vi "Test Step Parser.vi"(0 "Controller?":bool, 1 "LastDataTime":i64, 2 "Enum.Radio":enum32{"Flow", "Test", "Hot\nFuel"}(ring)=enum."Test", 5 "Step In":i32, 7 "CMD Cluster IN":T1, 9 "Profile":string[][](array[string]), 11 "Stable Count":dbl format="%#_13g", 12 "Parameter Timeout":dbl format="%#_13g") -> (3 "StepDataActive":dbl, 4 "StepTimeLimit":dbl, 6 "Step Out":i32, 8 "CMD Cluster Out":T1)   [LabVIEW 2019]
uses:
  TypeDef/Command Cluster.ctl
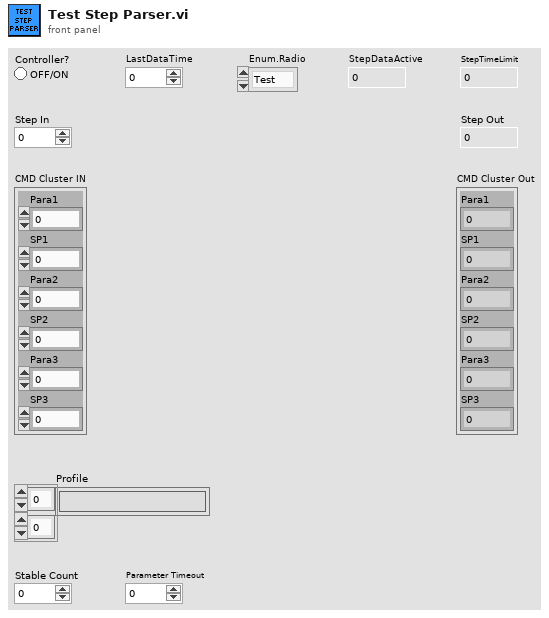
[diagram p1: front panel]
types:
  T1 = typedef "Command Cluster.ctl" = cluster{"Para1":i32, "SP1":dbl, "Para2":i32, "SP2":dbl, "Para3":i32, "SP3":dbl}
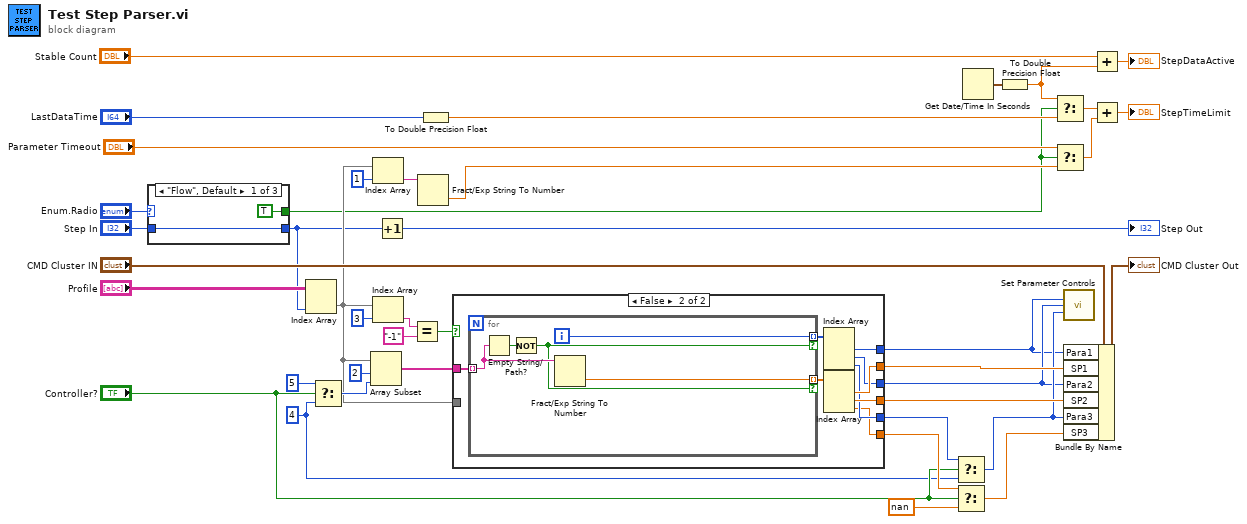
[diagram p0: block diagram]
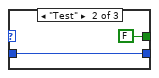
[diagram p2: hidden frame]
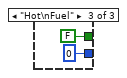
[diagram p3: hidden frame]
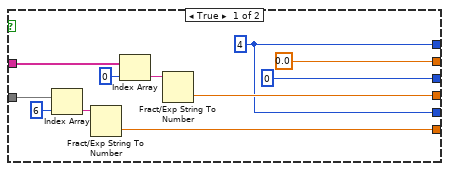
[diagram p4: hidden frame]
diagram:
  w24 = 4 ("index")
  n1 = case shown="\"Flow\", Default" "Enum.Radio" {
    tunnel: [TRUE FALSE FALSE] -> w1
    tunnel: "Step In" -> [w42 w44 _]
    tunnel: [w42 w44 0 ("Step In")] -> w2
    frame "Flow", Default {
    }
    frame "Test" {
    }
    frame "Hot\nFuel" {
    }
  }
  n2 = Index Array(array="Profile", index (col)=w2) -> (element=w19:string[])  [unwired: 1 in]
  n3 = Select(t=5 ("length"), s="Controller?", f=w24) -> (s? t:f=w29:i32)
  n4 = Array Subset(array=w19, index=2, length=w29) -> (w37:string[])
  n5 = Index Array(array=w19, index=1) -> (element=w17:string)
  n6 = Index Array(array=w19, index=3) -> (element=w33:string)
  n7 = Increment(x=w2) -> (x+1=→"Step Out":i32)
  n8 = Equal?(x=w33, y="-1") -> (x = y?=w31:bool)
  n9 = Fract/Exp String To Number(string=w17) -> (number=w13:dbl)  [unwired: 3 in, 1 out]
  n10 = To Double Precision Float(number="LastDataTime") -> (double precision float=w5:dbl)
  n11 = case shown="False" w31 {
    tunnel: w37 -> [w58 w67]
    tunnel: [0.0 w64] -> w36
    tunnel: [w55 w63] -> w35
    tunnel: [w52 w62] -> w20
    tunnel: [0 w61] -> w21
    tunnel: [w52 w60] -> w26
    tunnel: [w48 w59] -> w28
    tunnel: w19 -> [w49 _]
    frame True {
      w52 = 4
      n12 = Index Array(array=w49, index=6) -> (element=w50:string)
      n13 = Fract/Exp String To Number(string=w50) -> (number=w48:dbl)  [unwired: 3 in, 1 out]
      n14 = Index Array(array=w58, index=0) -> (element=w56:string)
      n15 = Fract/Exp String To Number(string=w56) -> (number=w55:dbl)  [unwired: 3 in, 1 out]
    }
    frame False {
      n16 = for {
        tunnel: w67 -> [w72] mode=indexing
        tunnel: [w68] -> w66 mode=indexing if=w69
        tunnel: [w70] -> w65 mode=indexing if=w69
        i -> [w70]
        n17 = Empty String/Path?(string/path=w72) -> (empty?=w71:bool)
        n18 = Not(x=w71) -> (.not. x?=w69:bool)
        n19 = Fract/Exp String To Number(string=w72) -> (number=w68:dbl)  [unwired: 3 in, 1 out]
      }
      n20 = Index Array(array=w65) -> (element #1=w62:i32, element #2=w61:i32, element #3=w60:i32)  [unwired: 3 in]
      n21 = Index Array(array=w66) -> (element #1=w64:dbl, element #2=w63:dbl, element #3=w59:dbl)  [unwired: 3 in]
    }
  }
  n22 = Select(t=w26, s="Controller?", f=w24) -> (s? t:f=w22:i32)
  n23 = Select(t=w28, s="Controller?", f=nan) -> (s? t:f=w25:dbl)
  n24 = Get Date/Time In Seconds() -> (seconds since 1Jan1904=w15:timestamp)
  n25 = To Double Precision Float(number=w15) -> (double precision float=w8:dbl)
  n26 = Select(t=w8, s=w1, f=w5) -> (s? t:f=w7:dbl)
  n27 = Select(t="Parameter Timeout", s=w1, f=w13) -> (s? t:f=w16:dbl)
  n28 = call "Set Parameter Controls.vi"("Para 1"=w20, "Para 2"=w21, "Para 3"=w22) -> ()  [unwired: 12 in, 1 out]
  n29 = Bundle By Name(cluster="CMD Cluster IN", "Para1"=w20, "SP1"=w36, "Para2"=w21, "SP2"=w35, "Para3"=w22, "SP3"=w25) -> (→"CMD Cluster Out":T1)
  n30 = Add(x="Stable Count", y=w8) -> (x+y=→"StepDataActive":dbl)
  n31 = Add(x=w7, y=w16) -> (x+y=→"StepTimeLimit":dbl)
